vi "set_double_check_moving_by_name.vi"(8 "error in (no error)":errorcluster, 9 "double check element":cluster{"1st check":bool, "2nd check":bool}, 10 "name":string, 11 "MotorSystem in":refnum<class "MotorSystem.lvclass">) -> (0 "error out":errorcluster, 3 "MotorSystem out":refnum<class "MotorSystem.lvclass">)   [LabVIEW 2016, in "MotionControl_UFO_3DOF.lvlib" / "MotorSystem.lvclass"]
uses:
  <userlib>/MotionControl_UFO_3DOF/MotorSystem/MotorSystem.lvclass
  <userlib>/MotionControl_UFO_3DOF/MotorSystem/MotorSystem.lvclass/MotorSystem.ctl
  <userlib>/MotionControl_UFO_3DOF/OneMotion/OneMotion.lvclass/OneMotion.ctl
  <userlib>/MotionControl_UFO_3DOF/StepMotor/StepMotor.lvclass/StepMotor.ctl
  <userlib>/MotionControl_UFO_3DOF/MotorSystem/get_motion_by_name.vi
  <userlib>/MotionControl_UFO_3DOF/StepMotor/set_moving.vi
  <userlib>/MotionControl_UFO_3DOF/OneMotion/get_StepMotor.vi
  <userlib>/MotionControl_UFO_3DOF/OneMotion/set_StepMotor.vi
  <userlib>/MotionControl_UFO_3DOF/MotorSystem/set_motion_by_name.vi
  <userlib>/MotionControl_UFO_3DOF/StepMotor/StepMotor.lvclass
  <userlib>/MotionControl_UFO_3DOF/OneMotion/OneMotion.lvclass
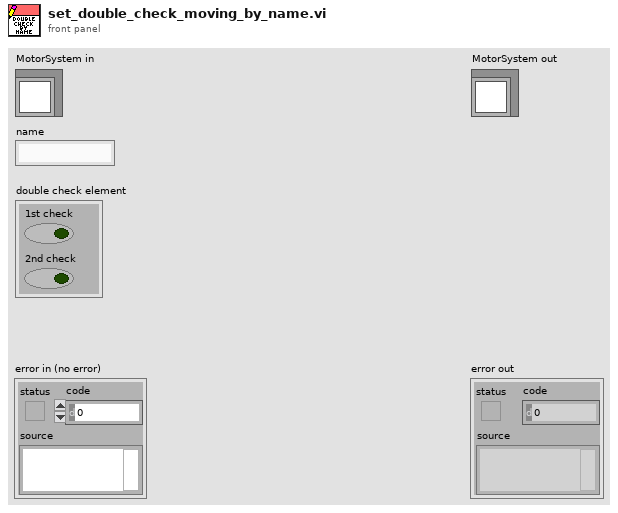
[diagram p1: front panel]
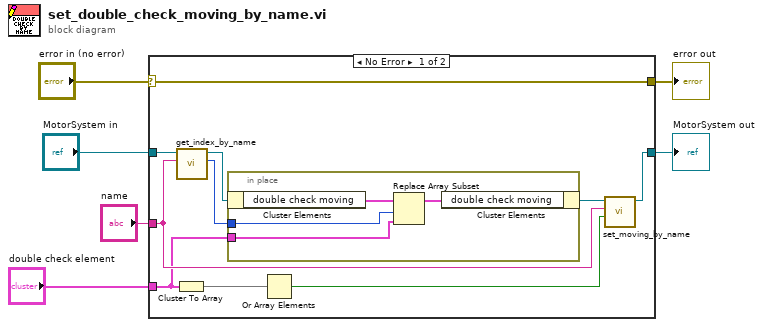
[diagram p0: block diagram]
diagram:
  n1 = case shown="No Error" "error in (no error)" {
    selector: "error in (no error)" -> [w16 w21]
    tunnel: [w16 w21] -> w5
    tunnel: [w11 w22] -> w3
    tunnel: "MotorSystem in" -> [w15 w22]
    tunnel: "double check element" -> [w9 _]
    tunnel: "name" -> [w10 _]
    frame No Error {
      n2 = Cluster To Array(cluster=w9) -> (array=w8:bool[])
      n3 = call <userlib>:"get_index_by_name.vi"("name"=w10, "MotorSystem 输入"=w15) -> ("index (0-based)"=w14:u32, "MotorSystem 输出"=w13:refnum<class "MotorSystem.lvclass">)  [unwired: 7 in, 1 out]
      n4 = in-place {
        in-place-border: w14 -> [w18]
        in-place-border: w9 -> [w17]
        n5 = in-place-cluster #1(w13) -> ("double check moving"=w20:cluster{"1st check":bool, "2nd check":bool}[])
        n6 = Replace Array Subset(array=w20, new element=w17, index=w18) -> (w19:cluster{"1st check":bool, "2nd check":bool}[])
        n7 = in-place-cluster #1("double check moving"=w19) -> (w12:refnum<class "MotorSystem.lvclass">)
      }
      n8 = Or Array Elements(Boolean array=w8) -> (logical OR=w7:bool)
      n9 = call <userlib>:"set_moving_by_name.vi"("moving?"=w7, "name"=w10, "MotorSystem输入"=w12) -> ("MotorSystem输出"=w11:refnum<class "MotorSystem.lvclass">)  [unwired: 7 in, 1 out]
    }
    frame Error {
    }
  }
  "error out" <- w5
  "MotorSystem out" <- w3
